vi "ep_Flicker Block4.vi"(0 "weighted voltage fluctuation":dbl[](array[numeric]), 1 "init":bool, 9 "input sampling rate":dbl=600.0) -> (4 "instant flicker":dbl[](array[numeric]))   [LabVIEW 2011, in "NI_EP_Power Quality.lvlib"]
doc: "This VI represents the squaring of the weighted flicker signal to simulate the non-linear eye-brain perception and the sliding mean averaging of the signal to simulate the storage effect in the brain (block 4 according IEC 61000-4-15)."
uses:
  <vilib>/addons/Electrical Power/PQ/NI_EP_Power Quality.lvlib
  <vilib>/Analysis/3filter.llb/Filter Passband Type.ctl
  <vilib>/Analysis/NI_AALBase.lvlib
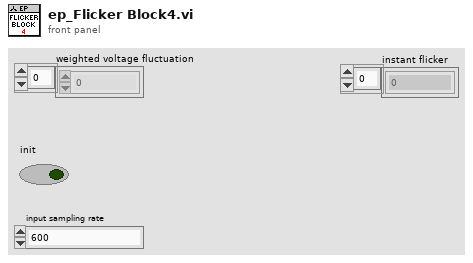
[diagram p1: front panel]
types:
  T1 = typedef "NI_AALBase.lvlib/Filter Passband Type.ctl" = enum32{"Lowpass", "Highpass", "Bandpass", "Bandstop"}
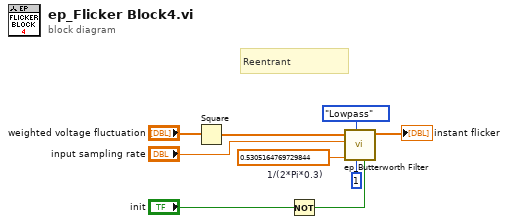
[diagram p0: block diagram]
diagram:
  w7 = 0.5305164769729844  # 1/(2*Pi*0.3)
  # "Reentrant"
  n1 = Square(x="weighted voltage fluctuation") -> (x^2=w1:dbl[])
  n2 = Not(x="init") -> (.not. x?=w9:bool)
  n3 = call <vilib>:"ep_Butterworth Filter.vi"("init/cont (init:F)"=w9, "order"=1, "filter type"=Filter_Passband_Type."Lowpass", "low cutoff freq: fl"=w7, "sampling freq: fs"="input sampling rate", "X"=w1) -> ("Filtered X"=→"instant flicker":dbl[])  [unwired: 4 in, 1 out]
